vi "ContainsFile.vi"(8 "error in (no error)":errorcluster, 10 "Path":path, 11 "Whitelist in":refnum<class "Whitelist.lvclass">) -> (0 "error out":errorcluster, 2 "Is Whitelisted?":bool, 3 "Whitelist out":refnum<class "Whitelist.lvclass">)   [LabVIEW 2019, in "Whitelist.lvclass"]
doc: "Returns true if the file is included in the whitelist."
uses:
  Whitelist.lvclass
  Whitelist.lvclass/Whitelist.ctl
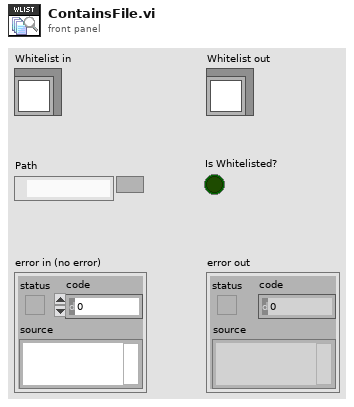
[diagram p1: front panel]
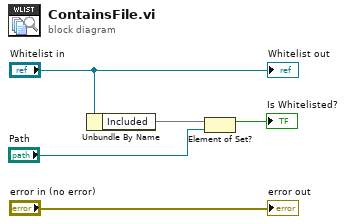
[diagram p0: block diagram]
diagram:
  n1 = Unbundle By Name("Whitelist in") -> ("Included"=w3:set{path})
  n2 = Element of Set?(10:"Path", 11:w3) -> (3:→"Is Whitelisted?":bool)
  "error out" <- "error in (no error)"
  "Whitelist out" <- "Whitelist in"
